vi "Get_Set_Account_Details.vi"(0 "Updated_Account_Details":string[][](array[string]), 11 "error in (no error)":errorcluster, 13 "File_Operation_Select":T1=enum."Update_Details") -> (4 "Account_Details":string[][](array[string]), 15 "error out":errorcluster)   [LabVIEW 2023]
doc: "Used to read and write the Account details form text file."
uses:
  Controls/File_Operation_Select.ctl
  <vilib>/Utility/file.llb/Read Delimited Spreadsheet (string).vi
  <vilib>/Utility/file.llb/Write Delimited Spreadsheet (string).vi
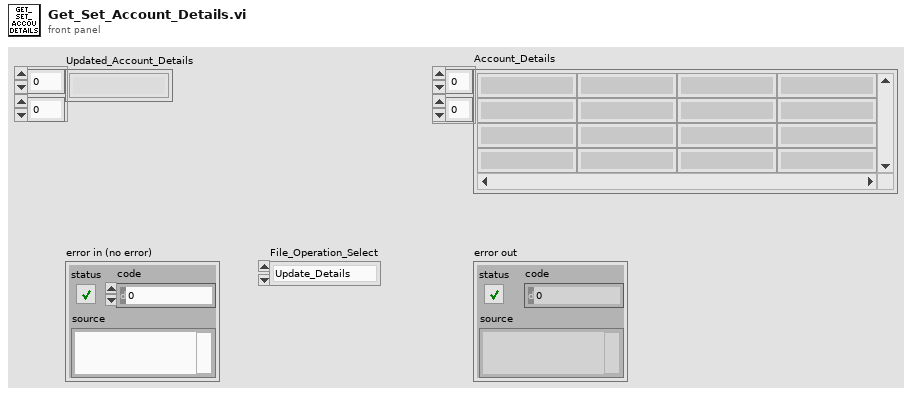
[diagram p1: front panel]
types:
  T1 = typedef "File_Operation_Select.ctl" = enum16{"Get_Details", "Update_Details"}
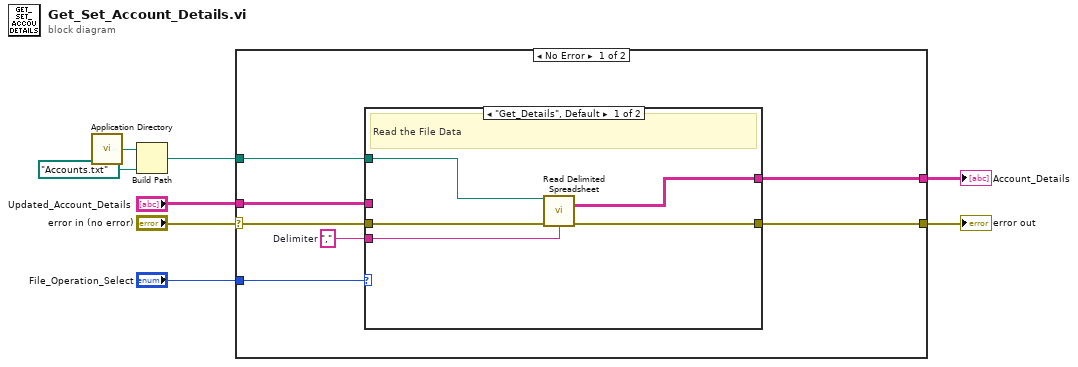
[diagram p0: block diagram]
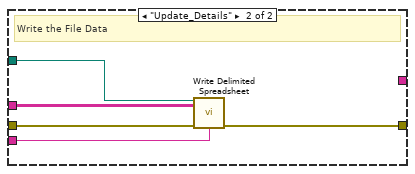
[diagram p2: hidden frame]
diagram:
  n1 = call <vilib>:"Application Directory.vi"() -> ("Application Directory"=w7:path)
  n2 = Build Path(base path=w7, name or relative path=path "Accounts.txt") -> (appended path=w6:path)
  n3 = case shown="No Error" "error in (no error)" {
    selector: "error in (no error)" -> [w13 w26]
    tunnel: w6 -> [w15 _]
    tunnel: [w14 w26] -> w5
    tunnel: "File_Operation_Select" -> [w12 _]
    tunnel: "Updated_Account_Details" -> [w10 _]
    tunnel: [w9 _] -> w1
    frame No Error {
      w11 = ","  # Delimiter
      n4 = case shown="\"Get_Details\", Default" w12 {
        tunnel: w15 -> [w20 w22]
        tunnel: [w19 w24] -> w14
        tunnel: w13 -> [w18 w25]
        tunnel: w11 -> [w17 w23]
        tunnel: w10 -> [_ w21]
        tunnel: [w16 _] -> w9
        frame "Get_Details", Default {
          # "Read the File Data"
          n5 = call-poly <vilib>:"Read Delimited Spreadsheet.vi"("file path (dialog if empty)"=w20, "error in (no error)"=w18, "delimiter (\\t)"=w17) -> ("all rows"=w16:string[][], "error out"=w19:errorcluster)  [unwired: 7 in, 4 out]
        }
        frame "Update_Details" {
          # "Write the File Data"
          n6 = call-poly <vilib>:"Write Delimited Spreadsheet.vi"("file path (dialog if empty)"=w22, "2D data"=w21, "error in (no error)"=w25, "delimiter (\\t)"=w23) -> ("error out"=w24:errorcluster)  [unwired: 10 in, 1 out]
        }
      }
    }
    frame Error {
    }
  }
  "error out" <- w5
  "Account_Details" <- w1
